vi "ep_Check Array Size (3x).vi"(8 "error in (no error)":errorcluster, 11 "number of channels":i32) -> (0 "error out":errorcluster, 3 "number of 3 phases":i32)   [LabVIEW 2014, in "NI_EP_Motor Monitoring.lvlib"]
uses:
  <vilib>/addons/Electrical Power/Motor Monitoring/NI_EP_Motor Monitoring.lvlib
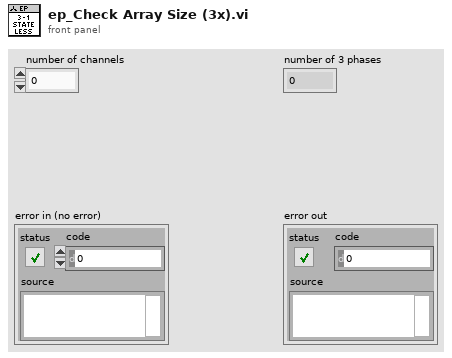
[diagram p1: front panel]
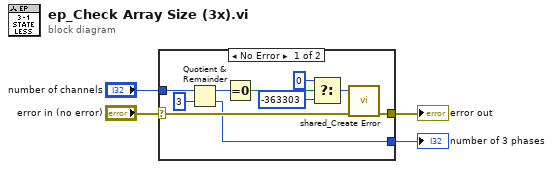
[diagram p0: block diagram]
diagram:
  n1 = case shown="No Error" "error in (no error)" {
    selector: "error in (no error)" -> [w8 w15]
    tunnel: [w7 w15] -> w3
    tunnel: "number of channels" -> [w6 _]
    tunnel: [w5 _] -> w1
    frame No Error {
      n2 = Quotient & Remainder(x=w6, y=3) -> (x-y*floor(x/y)=w10:i32, floor(x/y)=w5:i32)
      n3 = Equal To 0?(x=w10) -> (x = 0?=w13:bool)
      n4 = Select(t=0 ("error code (0)"), s=w13, f=-363303 ("error code (0)")) -> (s? t:f=w14:i32)
      n5 = call <vilib>:"shared_Create Error.vi"("error in (no error)"=w8, "error code (0)"=w14) -> ("error out"=w7:errorcluster)  [unwired: 9 in]
    }
    frame Error {
    }
  }
  "error out" <- w3
  "number of 3 phases" <- w1
